vi "sutter driver.vi"(4 "stop":bool, 5 "error in":errorcluster, 7 "Pos error":sgl[](array[numeric]), 8 "VISA resource name":refnum<visa-resource-name>) -> (0 "error out":errorcluster, 1 "Numeric":i32, 2 "Curent Position":dbl[](array[numeric]), 3 "Send Position":dbl[](array[numeric]))   [LabVIEW 2016]
uses:
  <vilib>/Instr/_visa.llb/VISA Configure Serial Port (Instr).vi
panel:
  out "output array":dbl[](array[numeric])
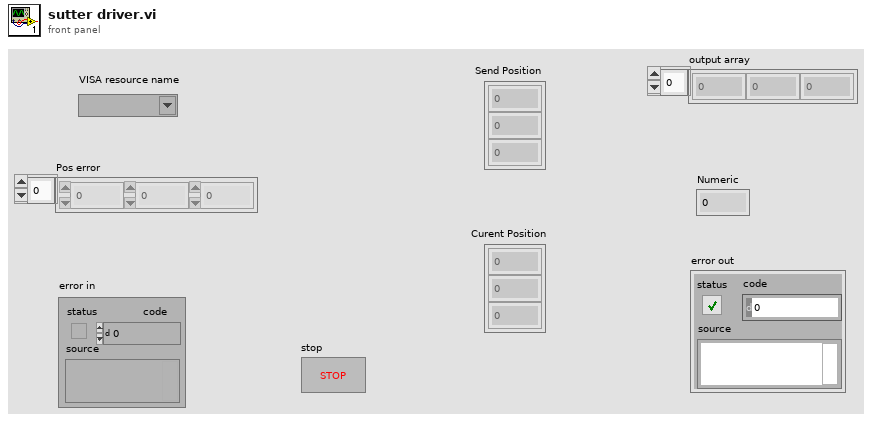
[diagram p1: front panel]
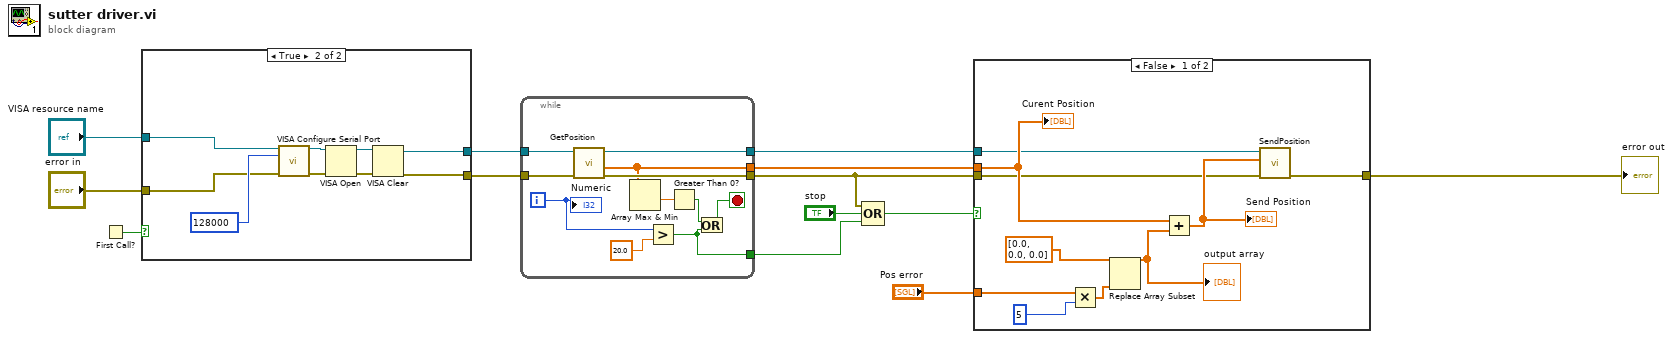
[diagram p0: block diagram]
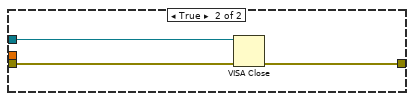
[diagram p2: hidden frame]
diagram:
  n1 = First Call?() -> (First Call?: T/F=w11:bool)
  n2 = case shown="True" w11 {
    tunnel: [w15 w19] -> w13
    tunnel: [w14 w18] -> w12
    tunnel: "VISA resource name" -> [w15 w17]
    tunnel: "error in" -> [w14 w16]
    frame False {
    }
    frame True {
      n3 = call-poly "VISA Configure Serial Port"("VISA resource name"=w17, "baud rate (9600)"=u32 128000, "error in (no error)"=w16) -> ("VISA resource name out"=w23:refnum<visa-resource-name>, "error out"=w22:errorcluster)  [unwired: 11 in]
      n4 = VISA Open(error in (no error)=w22, VISA resource name=w23) -> (VISA resource name=w21:refnum<visa-resource-name>, error out=w20:errorcluster)  [unwired: 3 in]
      n5 = VISA Clear(VISA resource name=w21, error in (no error)=w20) -> (VISA resource name out=w19:refnum<visa-resource-name>, error out=w18:errorcluster)
    }
  }
  n6 = while {
    tunnel: [w31] -> w3
    tunnel: w13 -> [w34]
    tunnel: [w33] -> w4
    tunnel: w12 -> [w35]
    tunnel: [w32] -> w2
    tunnel: [w25] -> w6
    i -> [w29]
    stop <- w26 stop-if-true
    n7 = call "GetPosition.vi"("error in"=w35, "VISA resource name in"=w34) -> ("error out"=w32:errorcluster, "Position XYZ"=w31:dbl[], "VISA resource name out"=w33:refnum<visa-resource-name>)  [unwired: 3 in, 1 out]
    n8 = Array Max & Min(array=w31) -> (min value=w28:dbl)  [unwired: 3 out]
    n9 = Greater?(x=w29, y=20.0) -> (0:w25:bool)
    n10 = Greater Than 0?(x=w28) -> (x > 0?=w27:bool)
    n11 = Or(x=w27, y=w25) -> (x .or. y?=w26:bool)
    "Numeric" <- w29
  }
  n12 = Compound Arithmetic op=OR(w2, "stop", w6) -> (w5:bool)
  n13 = case shown="False" w5 {
    tunnel: w4 -> [w39 w48]
    tunnel: w2 -> [w38 w47]
    tunnel: [w36 w46] -> w8
    tunnel: w3 -> [w40 _]
    tunnel: "Pos error" -> [w37 _]
    frame False {
      n14 = Multiply(x=w37, y=5 ("number: 0 to 1")) -> (x*y=w43:sgl[])
      n15 = Replace Array Subset(array=dbl[] [0.0, 0.0, 0.0], new element=w43) -> (w45:dbl[])  [unwired: 1 in]
      "output array" <- w45
      n16 = Add(x=w40, y=w45) -> (x+y=w42:dbl[])
      "Send Position" <- w42
      n17 = call "SendPosition.vi"("error in"=w38, "Motor Position"=w42, "VISA resource In"=w39) -> ("error out"=w36:errorcluster)  [unwired: 5 in, 1 out]
      "Curent Position" <- w40
    }
    frame True {
      n18 = VISA Close(VISA resource name=w48, error in (no error)=w47) -> (error out=w46:errorcluster)
    }
  }
  "error out" <- w8
